vi "Refresh.vi"(8 "error in":errorcluster, 10 "Attrs array in":T1[](array[typedef]), 11 "Ctrl array in":u32[](array[numeric])) -> (0 "error out":errorcluster, 2 "Attrs array out":T1[](array[typedef]), 3 "Ctrl array out":u32[](array[numeric]))   [LabVIEW 2012, in "Spinner.xctl"]
uses:
  Spinner.xctl
  Attrs.ctl
  Command.ctl
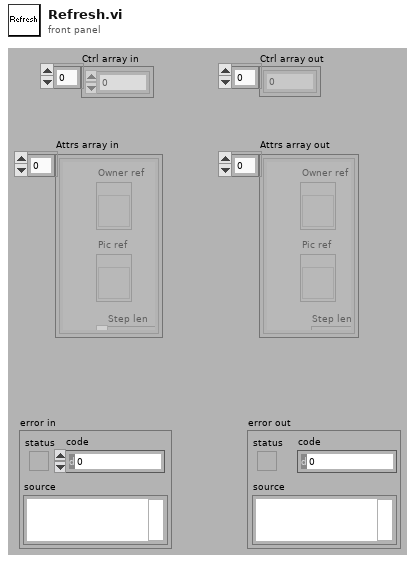
[diagram p1: front panel]
types:
  T1 = typedef "Spinner.xctl/Attrs.ctl" = cluster{"Owner ref":refnum<vi>, "Pic ref":refnum<vi>, "Step len":dbl, "Imgs":picture[], "Current phase":dbl}
  T2 = typedef "Spinner.xctl/Command.ctl" = enum16{"Add Control", "Remove Control", "Update Imgs", "Update Speed", "Refresh"}
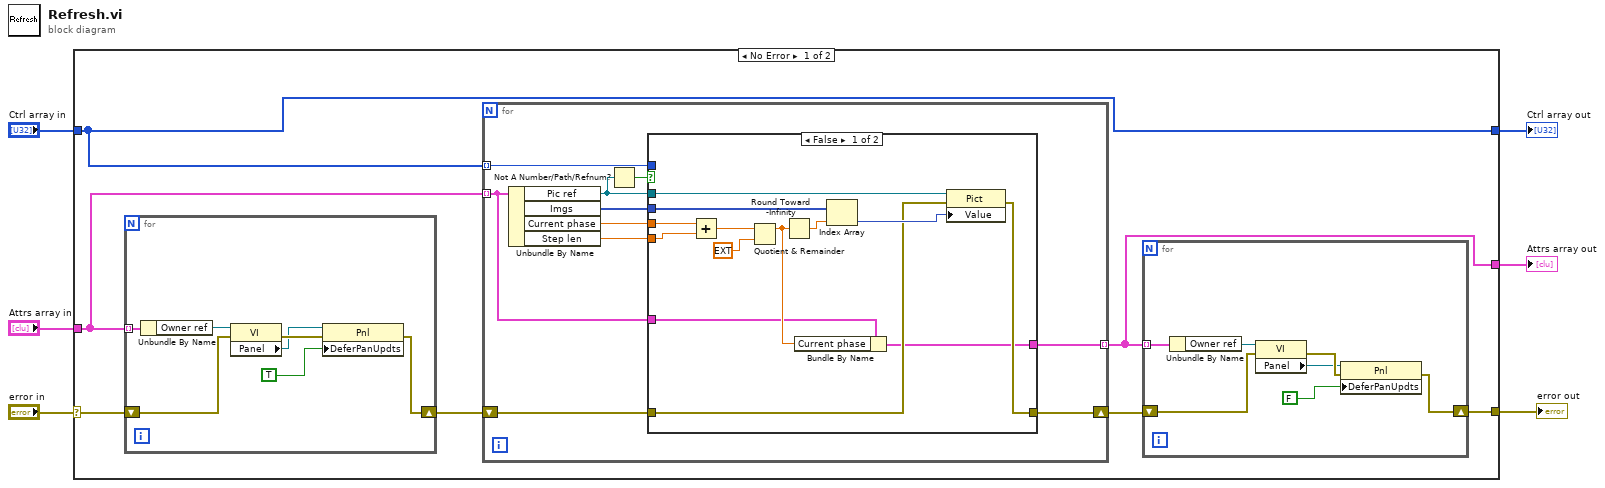
[diagram p0: block diagram]
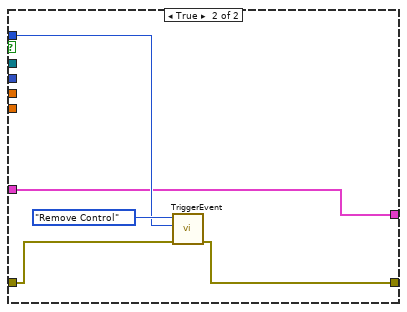
[diagram p2: hidden frame]
diagram:
  n1 = case shown="No Error" "error in" {
    selector: "error in" -> [w13 w56]
    tunnel: "Ctrl array in" -> [w10 w58]
    tunnel: "Attrs array in" -> [w11 w57]
    tunnel: [w8 w57] -> w4
    tunnel: [w10 w58] -> w3
    tunnel: [w7 w56] -> w1
    frame No Error {
      n2 = for {
        tunnel: w11 -> [w24] mode=indexing
        shift-right: [w21] -> w12
        shift-left: w13 -> [w22]
        n3 = Unbundle By Name(w24) -> ("Owner ref"=w23:refnum<vi>)
        n4 = property class="VI"(reference=w23, error in=w22) -> (error out=w27:errorcluster, "Panel"=w26:refnum<vi>)  [unwired: 1 out]
        n5 = property class="Pnl"(reference=w26, error in=w27, "DeferPanUpdts"=TRUE ("Defer Panel Updates")) -> (error out=w21:errorcluster)  [unwired: 1 out]
      }
      n6 = for {
        shift-right: [w30] -> w9
        shift-left: w12 -> [w35]
        tunnel: w11 -> [w29] mode=indexing
        tunnel: w10 -> [w36] mode=indexing
        tunnel: [w28] -> w8 mode=indexing
        n7 = Unbundle By Name(w29) -> ("Pic ref"=w31:refnum<vi>, "Imgs"=w34:picture[], "Current phase"=w33:dbl, "Step len"=w32:dbl)
        n8 = Not A Number/Path/Refnum?(number/path/refnum=w31) -> (NaN/Path/Refnum?=w37:bool)
        n9 = case shown="False" w37 {
          tunnel: w36 -> [_ w54]
          tunnel: w35 -> [w44 w53]
          tunnel: w34 -> [w47 _]
          tunnel: w33 -> [w43 _]
          tunnel: w32 -> [w42 _]
          tunnel: w31 -> [w46 _]
          tunnel: [w41 w51] -> w30
          tunnel: w29 -> [w39 w52]
          tunnel: [w38 w52] -> w28
          frame False {
            n10 = Add(x=w43, y=w42) -> (x+y=w49:dbl)
            n11 = Quotient & Remainder(x=w49, y=ext 30.0) -> (x-y*floor(x/y)=w40:ext)  [unwired: 1 out]
            n12 = Round Toward -Infinity(1:w40) -> (0:w50:ext)
            n13 = Bundle By Name(cluster=w39, "Current phase"=w40) -> (w38:T1)
            n14 = Index Array(array=w47, index=w50) -> (element=w45:picture)
            n15 = property class="Pict"(reference=w46, error in=w44, "Value"=w45) -> (error out=w41:errorcluster)  [unwired: 1 out]
          }
          frame True {
            n16 = call "TriggerEvent.vi"("error in"=w53, "Ctrl Ref"=w54, "Command"=Command."Remove Control") -> ("error out"=w51:errorcluster)  [unwired: 8 in]
          }
        }
      }
      n17 = for {
        shift-right: [w16] -> w7
        shift-left: w9 -> [w14]
        tunnel: w8 -> [w17] mode=indexing
        n18 = Unbundle By Name(w17) -> ("Owner ref"=w15:refnum<vi>)
        n19 = property class="VI"(reference=w15, error in=w14) -> (error out=w20:errorcluster, "Panel"=w19:refnum<vi>)  [unwired: 1 out]
        n20 = property class="Pnl"(reference=w19, error in=w20, "DeferPanUpdts"=FALSE ("Defer Panel Updates")) -> (error out=w16:errorcluster)  [unwired: 1 out]
      }
    }
    frame Error {
    }
  }
  "error out" <- w1
  "Attrs array out" <- w4
  "Ctrl array out" <- w3
